vi "Visa to File.vi"(0 "VISA resource name in":refnum<visa-resource-name>, 1 "Visa Error":errorcluster, 2 "Array in from shift reg":string[](array[string]), 3 "File data refnum":refnum<file>, 4 "File handle Error":errorcluster, 5 "Antenna offset":dbl max=0.0, 6 "UPDT COM switch":bool, 7 "Name of RCVR 1":string="RCVR 1" caption="Name of RCVR", 8 "Grennich Offset":dbl=-8.0) -> (11 "End Visa Loop":bool, 12 "Last 10 RCVR 1":string[](array[string]), 13 "End File Loop":bool, 14 "VISA resource name out":refnum<visa-resource-name>, 15 "Visa error out":errorcluster, 16 "Array out to shift reg":string[](array[string]), 17 "File data refnum out":refnum<file>, 18 "File Error out":errorcluster)   [LabVIEW 2011]
uses:
  <vilib>/Instr/_visa.llb/VISA Flush IO Buffer Mask.ctl
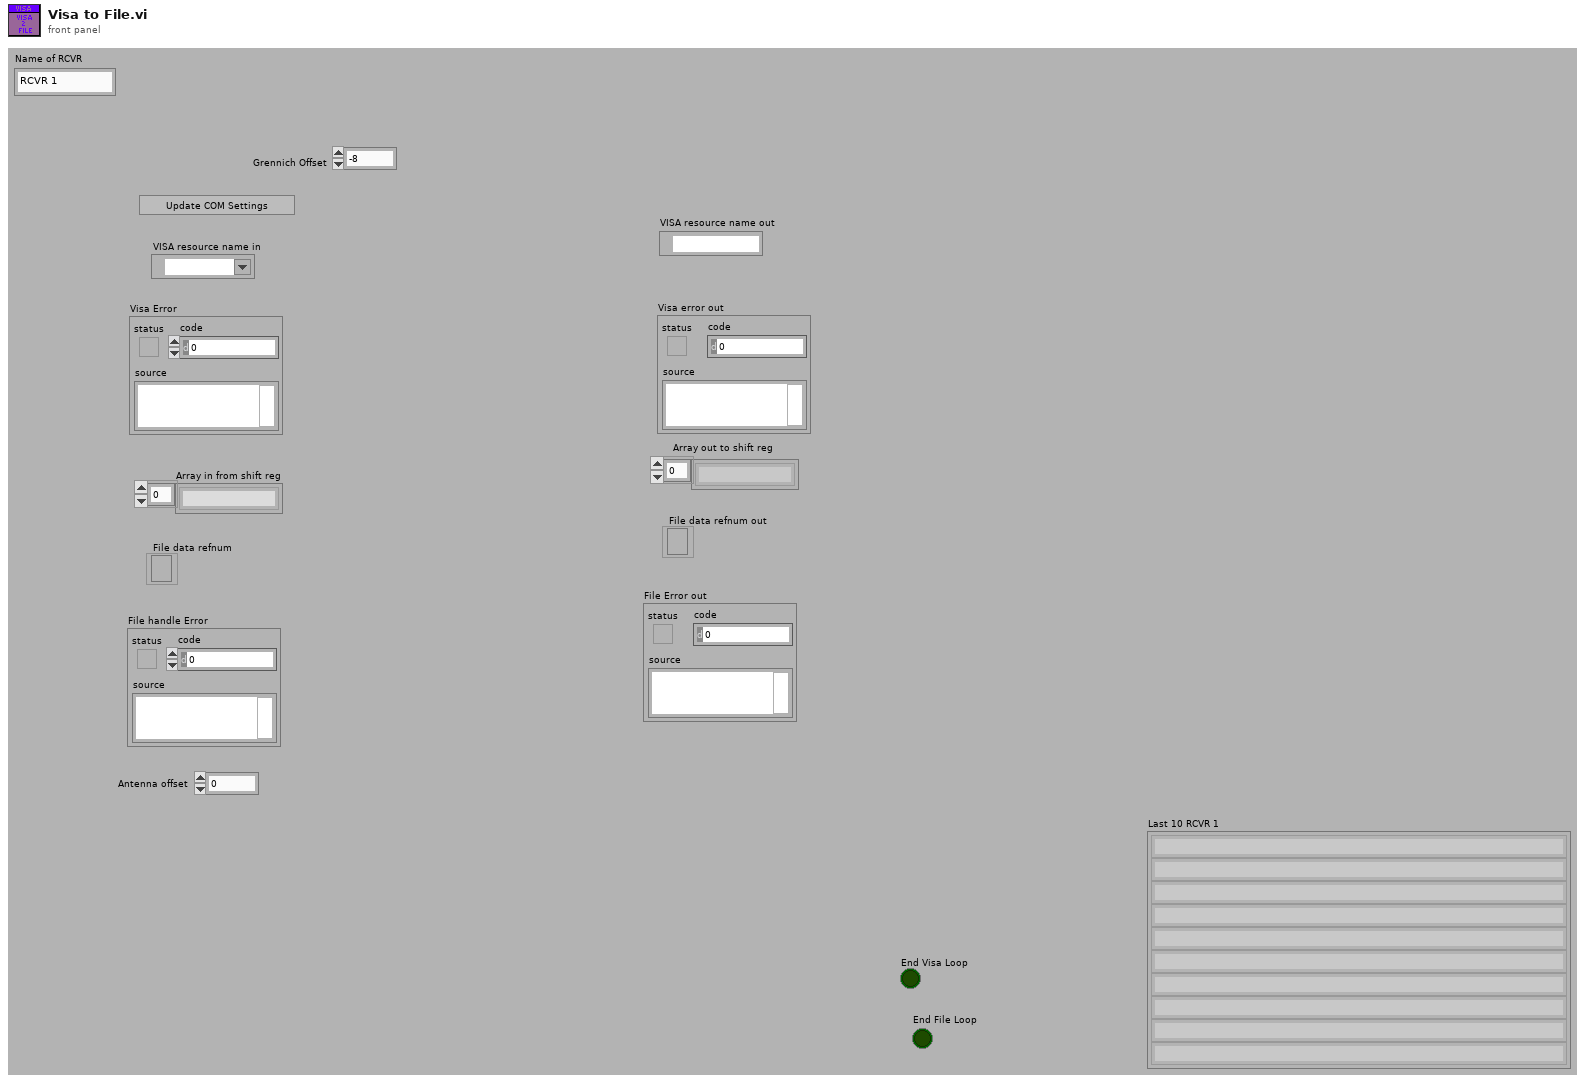
[diagram p1: front panel]
types:
  T1 = cluster{"Number of hours To Collect before starting new file ":u16, "Base File Path":path, "Update setup":bool, "Shutdown software":bool, "Time between samples (seconds)":u32}
  T2 = typedef "VISA Flush IO Buffer Mask.ctl" = u16
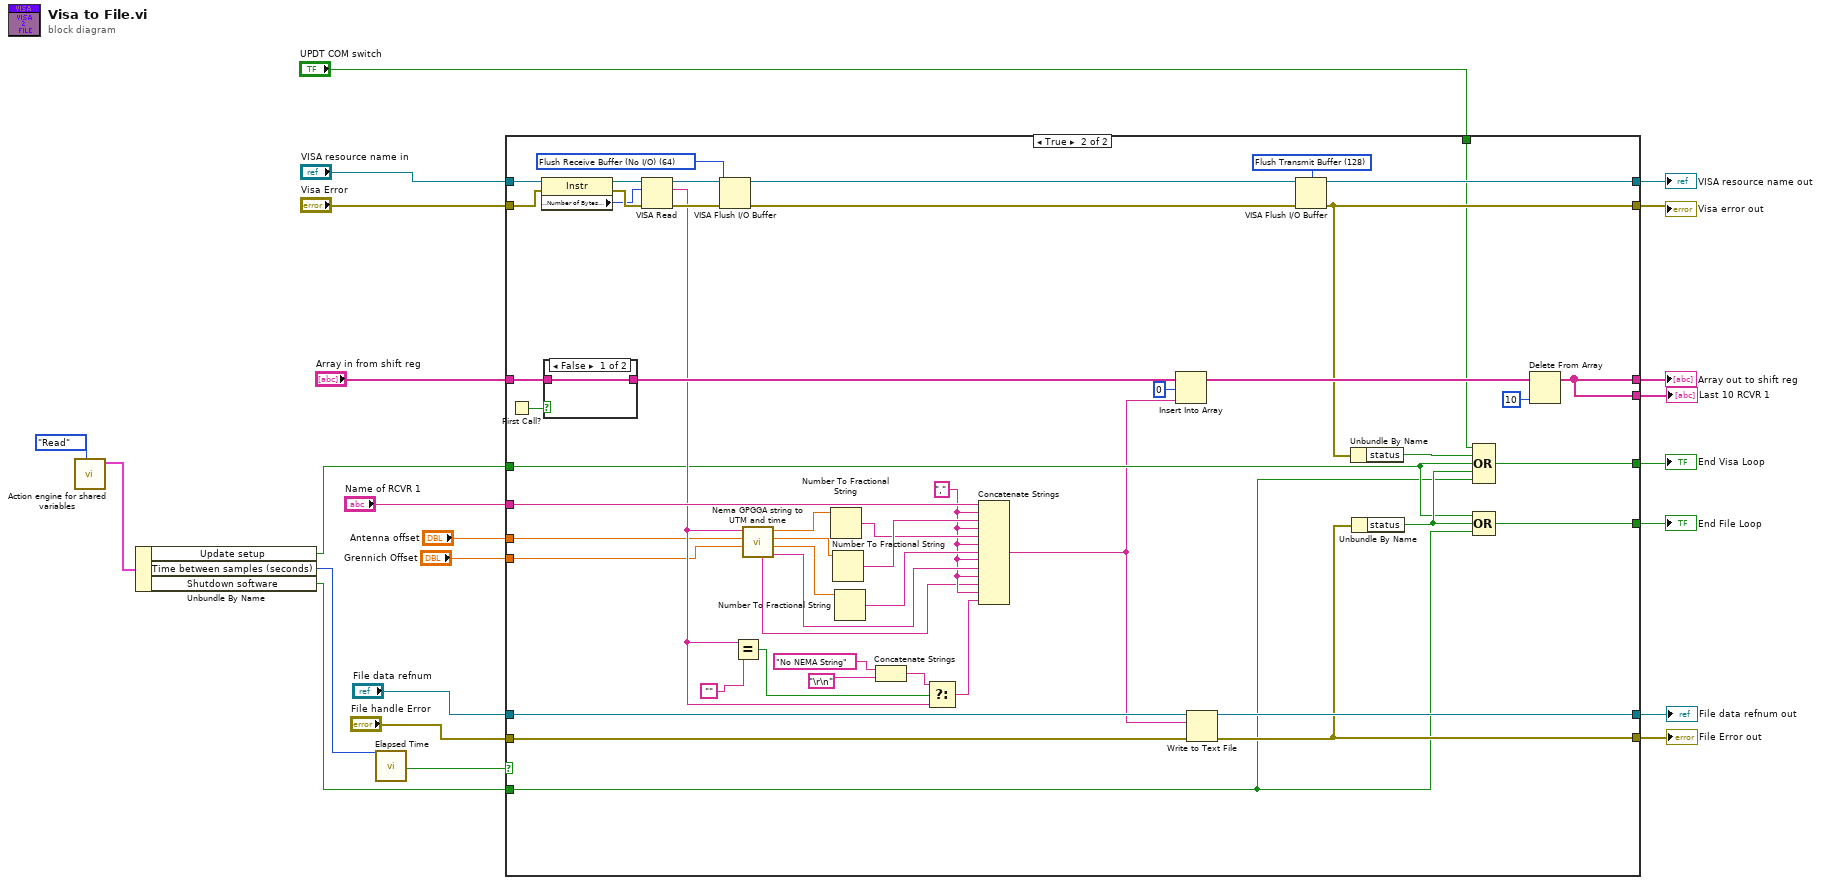
[diagram p0: block diagram]
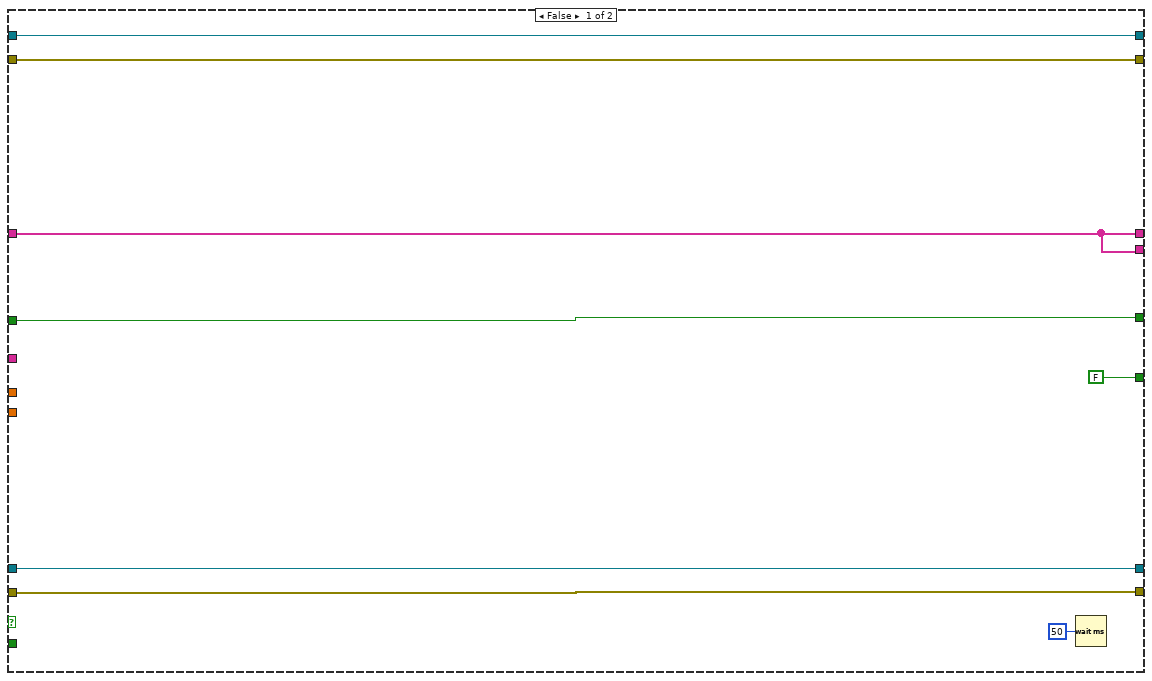
[diagram p2: hidden frame]
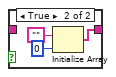
[diagram p3: hidden frame]
diagram:
  n1 = call "Action engine for shared variables.vi"("read/write"=enum16{"Read", "Write"}."Read") -> ("func global variables read"=w4:T1)  [unwired: 9 in, 1 out]
  n2 = Unbundle By Name(w4) -> ("Update setup"=w9:bool, "Time between samples (seconds)"=w3:u32, "Shutdown software"=w8:bool)
  n3 = call "Elapsed Time"("Time Target (s)"=w3) -> ("Time has Elapsed"=w10:bool)  [unwired: 11 in, 7 out]
  n4 = case shown="True" w10 {
    tunnel: [w31 w66] -> w17
    tunnel: "VISA resource name in" -> [w31 w82]
    tunnel: "Visa Error" -> [w30 w81]
    tunnel: "File data refnum" -> [w29 w77]
    tunnel: [w29 w76] -> w12
    tunnel: "File handle Error" -> [w28 w75]
    tunnel: [w30 w59] -> w16
    tunnel: [w24 w74] -> w14
    tunnel: [w28 w57] -> w11
    tunnel: [FALSE w73] -> w13
    tunnel: [w25 w54] -> w15
    tunnel: "Array in from shift reg" -> [w25 w60]
    tunnel: w9 -> [w24 w36]
    tunnel: w8 -> [_ w35]
    tunnel: "UPDT COM switch" -> [_ w55]
    tunnel: [w25 w54] -> w7
    tunnel: "Name of RCVR 1" -> [_ w51]
    tunnel: "Antenna offset" -> [_ w33]
    tunnel: "Grennich Offset" -> [_ w32]
    frame False {
      n5 = Wait (ms)(milliseconds to wait=u32 50) -> ()  [unwired: 1 out]
    }
    frame True {
      w45 = "," ("string")
      w67 = T2 128 items=["Flush Receive Buffer"=16, "Write Transmit Buffer to Device"=32, "Flush Receive Buffer (No I/O)"=64, "Flush Transmit Buffer"=128] ("Mask")
      w68 = T2 64 items=["Flush Receive Buffer"=16, "Write Transmit Buffer to Device"=32, "Flush Receive Buffer (No I/O)"=64, "Flush Transmit Buffer"=128] ("Mask")
      n6 = First Call?() -> (First Call?: T/F=w65:bool)
      n7 = property class="Instr"(reference=w82, error in=w81) -> (reference out=w80:refnum<visa-resource-name>, error out=w79:errorcluster, "Serial Settings:Number of Bytes at Serial Port"=w78:u32)
      n8 = case shown="False" w65 {
        tunnel: [w83 w84] -> w64
        tunnel: w60 -> [w83 _]
        frame False {
        }
        frame True {
          n9 = Initialize Array("", 0 ("dimension size")) -> (w84:string[])
        }
      }
      n10 = VISA Read(VISA resource name=w80, byte count=w78, error in (no error)=w79) -> (VISA resource name out=w72:refnum<visa-resource-name>, read buffer=w42:string, error out=w71:errorcluster)  [unwired: 1 out]
      n11 = VISA Flush I/O Buffer(VISA resource name=w72, mask (16)=w68, error in (no error)=w71) -> (VISA resource name out=w69:refnum<visa-resource-name>, error out=w70:errorcluster)
      n12 = Equal?(x=w42, y="") -> (x = y?=w41:bool)
      n13 = call "Nema GPGGA string to UTM and time.vi"("Grennich Offset"=w32, "Antenna offset"=w33, "String In (NEAMA GGA)"=w42) -> ("date/time string"=w46:string, "Elevation"=w48:dbl, "Easting (M)"=w49:dbl, "Northing (M)"=w50:dbl, "Zone (string)"=w44:string)  [unwired: 4 in]
      n14 = Number To Fractional String(number=w50) -> (F-format string=w52:string)  [unwired: 3 in]
      n15 = Number To Fractional String(number=w49) -> (F-format string=w53:string)  [unwired: 3 in]
      n16 = Number To Fractional String(number=w48) -> (F-format string=w47:string)  [unwired: 3 in]
      n17 = Concatenate Strings("No NEMA String" ("string"), "\r\n") -> (w38:string)
      n18 = Select(t=w38, s=w41, f=w42) -> (s? t:f=w40:string)
      n19 = Concatenate Strings(w51, w45, w53, w45, w52, w45, w47, w45, w46, w45, w44, w45, w40) -> (w34:string)
      n20 = Insert Into Array(array=w64, index=0, new element=w34) -> (w62:string[])
      n21 = Write to Text File(file (use dialog)=w77, text=w34, error in=w75) -> (refnum out=w76:refnum<file>, error out=w57:errorcluster)  [unwired: 1 in, 1 out]
      n22 = VISA Flush I/O Buffer(VISA resource name=w69, mask (16)=w67, error in (no error)=w70) -> (VISA resource name out=w66:refnum<visa-resource-name>, error out=w59:errorcluster)
      n23 = Unbundle By Name(w59) -> ("status"=w58:bool)
      n24 = Unbundle By Name(w57) -> ("status"=w56:bool)
      n25 = Compound Arithmetic op=OR(w55, w58, w36, w56, w35) -> (w74:bool)
      n26 = Compound Arithmetic op=OR(w36, w56, w35) -> (w73:bool)
      n27 = Delete From Array(array=w62, index=10) -> (array with subset deleted=w54:string[])  [unwired: 1 in, 1 out]
    }
  }
  "VISA resource name out" <- w17
  "Visa error out" <- w16
  "Array out to shift reg" <- w15
  "End Visa Loop" <- w14
  "End File Loop" <- w13
  "File data refnum out" <- w12
  "File Error out" <- w11
  "Last 10 RCVR 1" <- w7
